vi "CalibMatrix (SubVI).vi"(0 "Calibration Files":path[](array[path])) -> (1 "Calib Matrix":dbl[][](array[numeric]), 2 "error out":errorcluster)   [LabVIEW 2021]
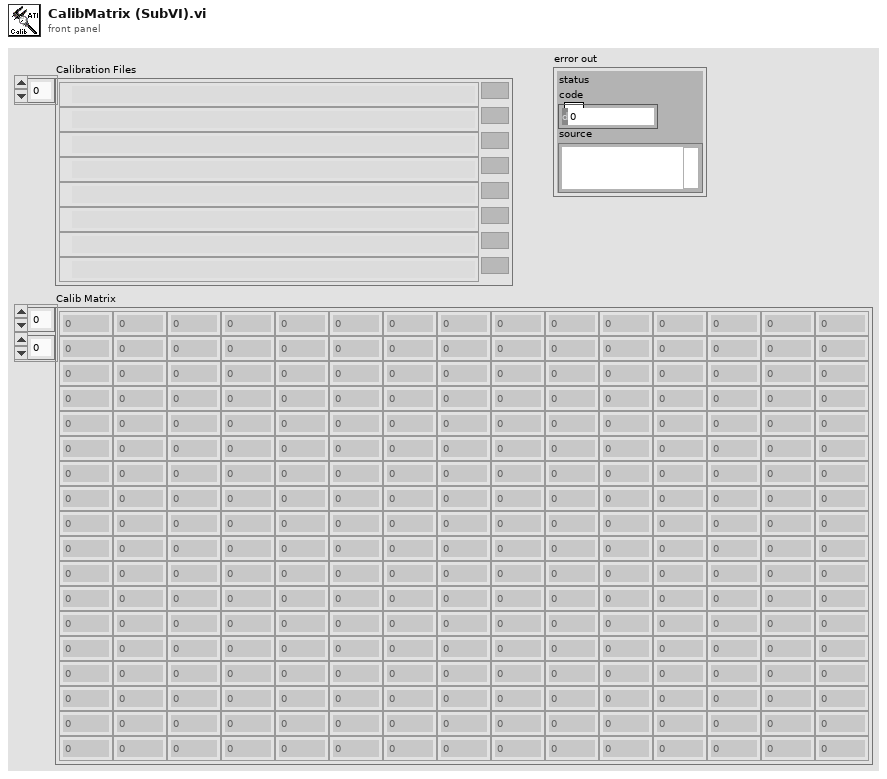
[diagram p1: front panel]
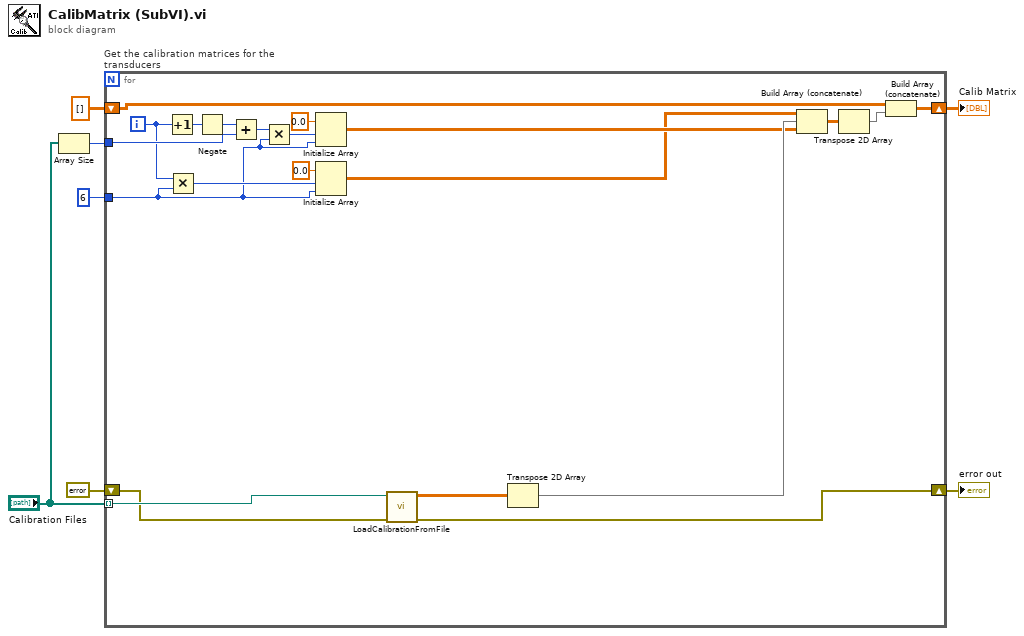
[diagram p0: block diagram]
diagram:
  n1 = Array Size(array="Calibration Files") -> (size(s)=w6:i32)
  n2 = for "Get the calibration matrices for the transducers" {
    tunnel: "Calibration Files" -> [w28] mode=indexing
    shift-right: [w27] -> w1
    shift-left: errorcluster {"status"=FALSE, "code"=0, "source"=""} ("error out") -> [w26]
    tunnel: 6 ("y") -> [w11]
    tunnel: w6 -> [w21]
    shift-right: [w9] -> w7
    shift-left: dbl[][] [] -> [w10]
    i -> [w20]
    n3 = Increment(x=w20) -> (x+1=w23:i32)
    n4 = Multiply(x=w20, y=w11) -> (x*y=w13:i32)
    n5 = Negate(x=w23) -> (-x=w22:i32)
    n6 = Add(x=w22, y=w21) -> (x+y=w12:i32)
    n7 = Multiply(x=w12, y=w11) -> (x*y=w14:i32)
    n8 = Initialize Array(0.0 ("element"), w14, w11) -> (w16:dbl[][])
    n9 = Initialize Array(0.0 ("element"), w13, w11) -> (w15:dbl[][])
    n10 = call "LoadCalibrationFromFile.vi"("Error In"=w26, "Cal File Path"=w28) -> ("Error Out"=w27:errorcluster, "Calibration Matrix"=w8:dbl[][])  [unwired: 2 in, 2 out]
    n11 = Transpose 2D Array(2D array=w8) -> (transposed array=w18:dbl[][])
    n12 = Build Array (concatenate)(w15, w18, w16) -> (w19:dbl[][])
    n13 = Transpose 2D Array(2D array=w19) -> (transposed array=w17:dbl[][])
    n14 = Build Array (concatenate)(w10, w17) -> (w9:dbl[][])
  }
  "Calib Matrix" <- w7
  "error out" <- w1
